vi "EnteringState.vi"(1 "IFw session":refnum<class "niInstr FIFO Register Bus v1 Host.lvclass">, 2 "FPGA Ref":refnum<k20>, 5 "Parameters":T4, 7 "StateIn":T1, 11 "error in (no error)":errorcluster) -> (8 "StateOut":T1, 15 "error out":errorcluster)   [LabVIEW 2017, in "AppStateMachine runtime.lvclass"]
uses:
  AppStateMachine runtime.lvclass
  <instrlib>/_niInstr/FIFO Register Bus/v1/Host/niInstr FIFO Register Bus v1 Host.lvclass
  parameter user data.ctl
  State.ctl
  StateId.ctl
  LED_Color.ctl
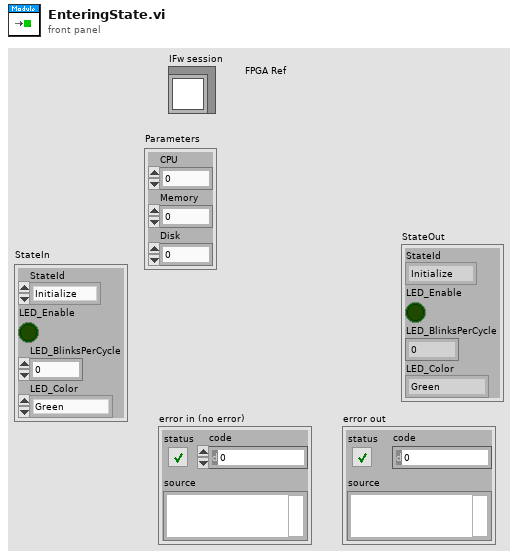
[diagram p1: front panel]
types:
  T1 = typedef "AppStateMachine runtime.lvclass/State.ctl" = cluster{"StateId":T2, "LED_Enable":bool, "LED_BlinksPerCycle":i32, "LED_Color":T3}
  T2 = typedef "AppStateMachine runtime.lvclass/StateId.ctl" = enum16{"Initialize", "Idle", "SafeState", "UnrecoverableSafeState"}
  T3 = typedef "AppStateMachine runtime.lvclass/LED_Color.ctl" = enum16{"Green", "Yellow"}
  T4 = typedef "AppStateMachine runtime.lvclass/parameter user data.ctl" = cluster{"CPU":dbl, "Memory":dbl, "Disk":dbl}
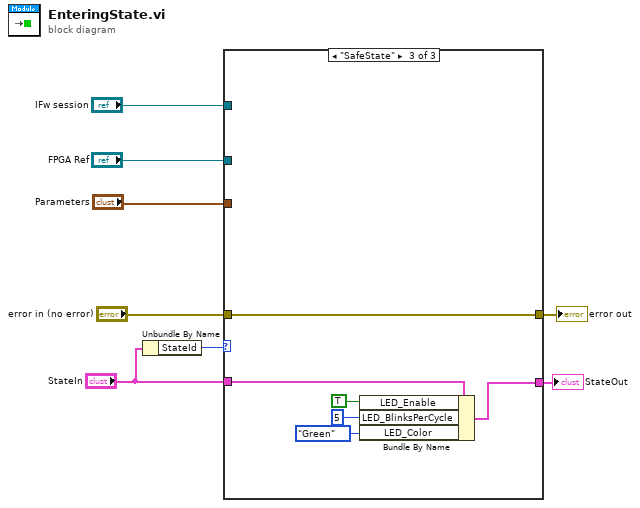
[diagram p0: block diagram]
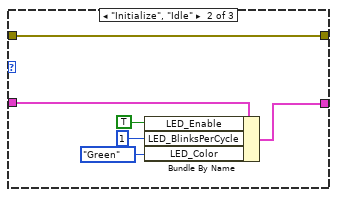
[diagram p3: hidden frame]
diagram:
  n1 = Unbundle By Name("StateIn") -> ("StateId"=w3:T2)
  n2 = case shown="\"SafeState\"" w3 {
    tunnel: "error in (no error)" -> [w10 w16 w22]
    tunnel: [w10 w16 w22] -> w8
    tunnel: "Parameters" -> [_ _ _]
    tunnel: "IFw session" -> [_ _ _]
    tunnel: "FPGA Ref" -> [_ _ _]
    tunnel: "StateIn" -> [w9 w15 w21]
    tunnel: [w9 w11 w17] -> w1
    frame Default {
    }
    frame "Initialize", "Idle" {
      n3 = Bundle By Name(cluster=w15, "LED_Enable"=TRUE, "LED_BlinksPerCycle"=1, "LED_Color"=LED_Color."Green") -> (w11:T1)
    }
    frame "SafeState" {
      n4 = Bundle By Name(cluster=w21, "LED_Enable"=TRUE, "LED_BlinksPerCycle"=5, "LED_Color"=LED_Color."Green") -> (w17:T1)
    }
  }
  "error out" <- w8
  "StateOut" <- w1
